vi "IMAQController.contents.vi"() -> ()   [LabVIEW 2014, in "IMAQController.lvlib"]
uses:
  IMAQController.lvlib
panel:
  out "error out":errorcluster
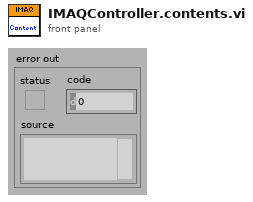
[diagram p1: front panel]
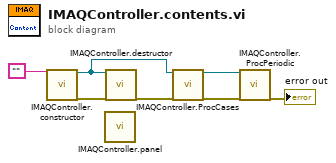
[diagram p0: block diagram]
diagram:
  n1 = call "IMAQController.constructor.vi"("name"="") -> ("i ref out"=w1:refnum<vi>, "error out"=w7:errorcluster)  [unwired: 16 in, 1 out]
  n2 = call "IMAQController.panel.vi"() -> ()  [unwired: 20 in]
  n3 = call "IMAQController.destructor.vi"("i ref in"=w1, "error in (no error)"=w7) -> ("error out"=w4:errorcluster)  [unwired: 17 in]
  n4 = call "IMAQController.ProcCases.vi"("i ref in"=w1, "error in (no error)"=w4) -> ("i ref out"=w6:refnum<vi>, "error out"=w5:errorcluster)  [unwired: 15 in, 1 out]
  n5 = call "IMAQController.ProcPeriodic.vi"("i ref in"=w6, "error in (no error)"=w5) -> ("error out"=→"error out":errorcluster)  [unwired: 15 in, 2 out]
